vi "Set Blinking Status.vi"(10 "data in":T1, 11 "Control in":refnum<vi>) -> (3 "Control out":refnum<vi>)   [LabVIEW 2020]
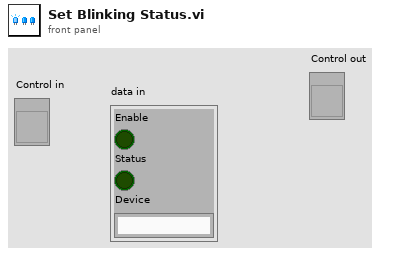
[diagram p1: front panel]
types:
  T1 = cluster{"Enable":bool, "Status":bool, "Device":string}
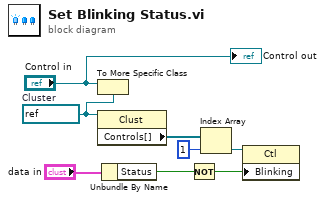
[diagram p0: block diagram]
diagram:
  w5 = refnum<vi> refnum  # Cluster
  n1 = To More Specific Class(target class=w5, reference="Control in") -> ()  [unwired: 1 in, 2 out]
  n2 = property class="Clust"(reference=w5) -> ("Controls[]"=w6:refnum<vi>[])  [unwired: 1 in, 2 out]
  n3 = Unbundle By Name("data in") -> ("Status"=w2:bool)
  n4 = Not(x=w2) -> (.not. x?=w1:bool)
  n5 = Index Array(array=w6, index=1) -> (element=w8:refnum<vi>)
  n6 = property class="Ctl"(reference=w8, "Blinking"=w1) -> ()  [unwired: 1 in, 2 out]
  "Control out" <- "Control in"
